vi "Find Average Center.vi"(5 "Position":i32, 7 "Tray Number":i32, 8 "Type of Hexaboard":T1, 9 "XYZTheta":dbl[](array[numeric]), 11 "Gantry In":refnum<k24>) -> (1 "XYZTheta":dbl[](array[numeric]) format="%.6g", 3 "Gantry Out":refnum<k24>)   [LabVIEW 2021, in "Component Tray.lvclass"]
uses:
  Component Tray.lvclass
  Find Component.ctl
  Controller/Camera/Machine Vision.ctl
  C:/Program Files (x86)/Aerotech/A3200/LabVIEW/2010/Bin/Aerotech.A3200.dll
  Program Files (x86)/Aerotech/A3200/LabVIEW/2010/Bin/Aerotech.A3200.dll
  Controller/Camera/Image processing.ctl
  Controller/Camera/Camera settings.ctl
  Controller/Camera/Material.ctl
  Routine/TypeOfHexaboard.ctl
  Controller/Camera/Edmund Optics/Edmund Optics.lvclass
  C:/Users/hep/Documents/UCSB-CMU-GantryCode/UCSB-Gantry-HEP-main (3)/UCSB-Gantry-HEP-main/Classes/Controller/Camera/Camera.lvclass
  Program Files (x86)/National Instruments/LabVIEW 2021/examples/Connectivity/Python/support/PythonVersionsEnum.ctl
  Controller/Camera/Camera.lvclass
  Controller/Motion/A3200/A3200.lvclass
  Controller/Motion/Motion.lvclass
  Routine/Routine.lvclass
panel:
  out "Program Stopped":bool
  out "XY Graph":cluster{"X":dbl, "Y":dbl}[](graph)
  out "Sensor ID Location":dbl[](array[numeric])
  in  "Go to Sensor ID":bool
  out "CH1 Location":dbl[](array[numeric])
  in  "Verify CH1":bool
  out "CH1 correct?":bool
  in  "Go to CH1":bool
  in  "Focus step size":dbl format="%#_13g"
  in  "number of focus steps":i32
  out "Average Strength":dbl
  in  "Focus":bool
  in  "Material":T2
  out "All fiducials recorded":bool
  in  "Override presets":bool
  in  "Camera settings":T3={"Gamma"=1.6, "Gain"=0, "Sharpness"=0, "Contrast"=0.0, "Exposure"=0.0078125} {"Exposure" min=0.000244140625 max=0.5 scale=0.0002..0.5; "Contrast" min=0.0 max=1.0 scale=0.001..1.0; "Sharpness" min=0 max=2 step=1 scale=0.0..2.0; "Gain" min=0 max=100 step=1 scale=0.1..100.0; "Gamma" min=0.01 max=10.0 scale=0.01..10.0}
  in  "Image processing":T4={"Brightness"=128.0, "Contrast"=45.0, "Gamma"=1.0471123} {"Brightness" scale=0.0..400.0; "Contrast" scale=0.0..90.0; "Gamma" scale=0.005..5.0}
  in  "Machine Vision":T5=enum."Sensor Fiducials"
  out "Gantry":dbl[](array[numeric]) format="%.6g"
  out "Sum":dbl[](array[numeric]) format="%.6g"
  out "Bottom Right XY":dbl[](array[numeric]) format="%.6g"
  out "Bottom Left XY":dbl[](array[numeric]) format="%.6g"
  out "Top Right XY":dbl[](array[numeric]) format="%.6g"
  out "Top Left XY":dbl[](array[numeric]) format="%.6g"
  in  "Record Bottom Left":bool
  in  "Record Bottom Right":bool
  in  "Record Top Right":bool
  in  "Record Top Left":bool
  in  "Go to Bottom Right":bool
  in  "Go to Bottom Left":bool
  in  "Go to Top Right":bool
  in  "Go to Top Left":bool
  in  "Joystick":bool
  out "Camera":dbl[](array[numeric]) format="%.6g"
  in  "Go to Center":bool
  in  "Component":T6
  in  "Stop Program":bool
  out "Image":T7(plugin-control)
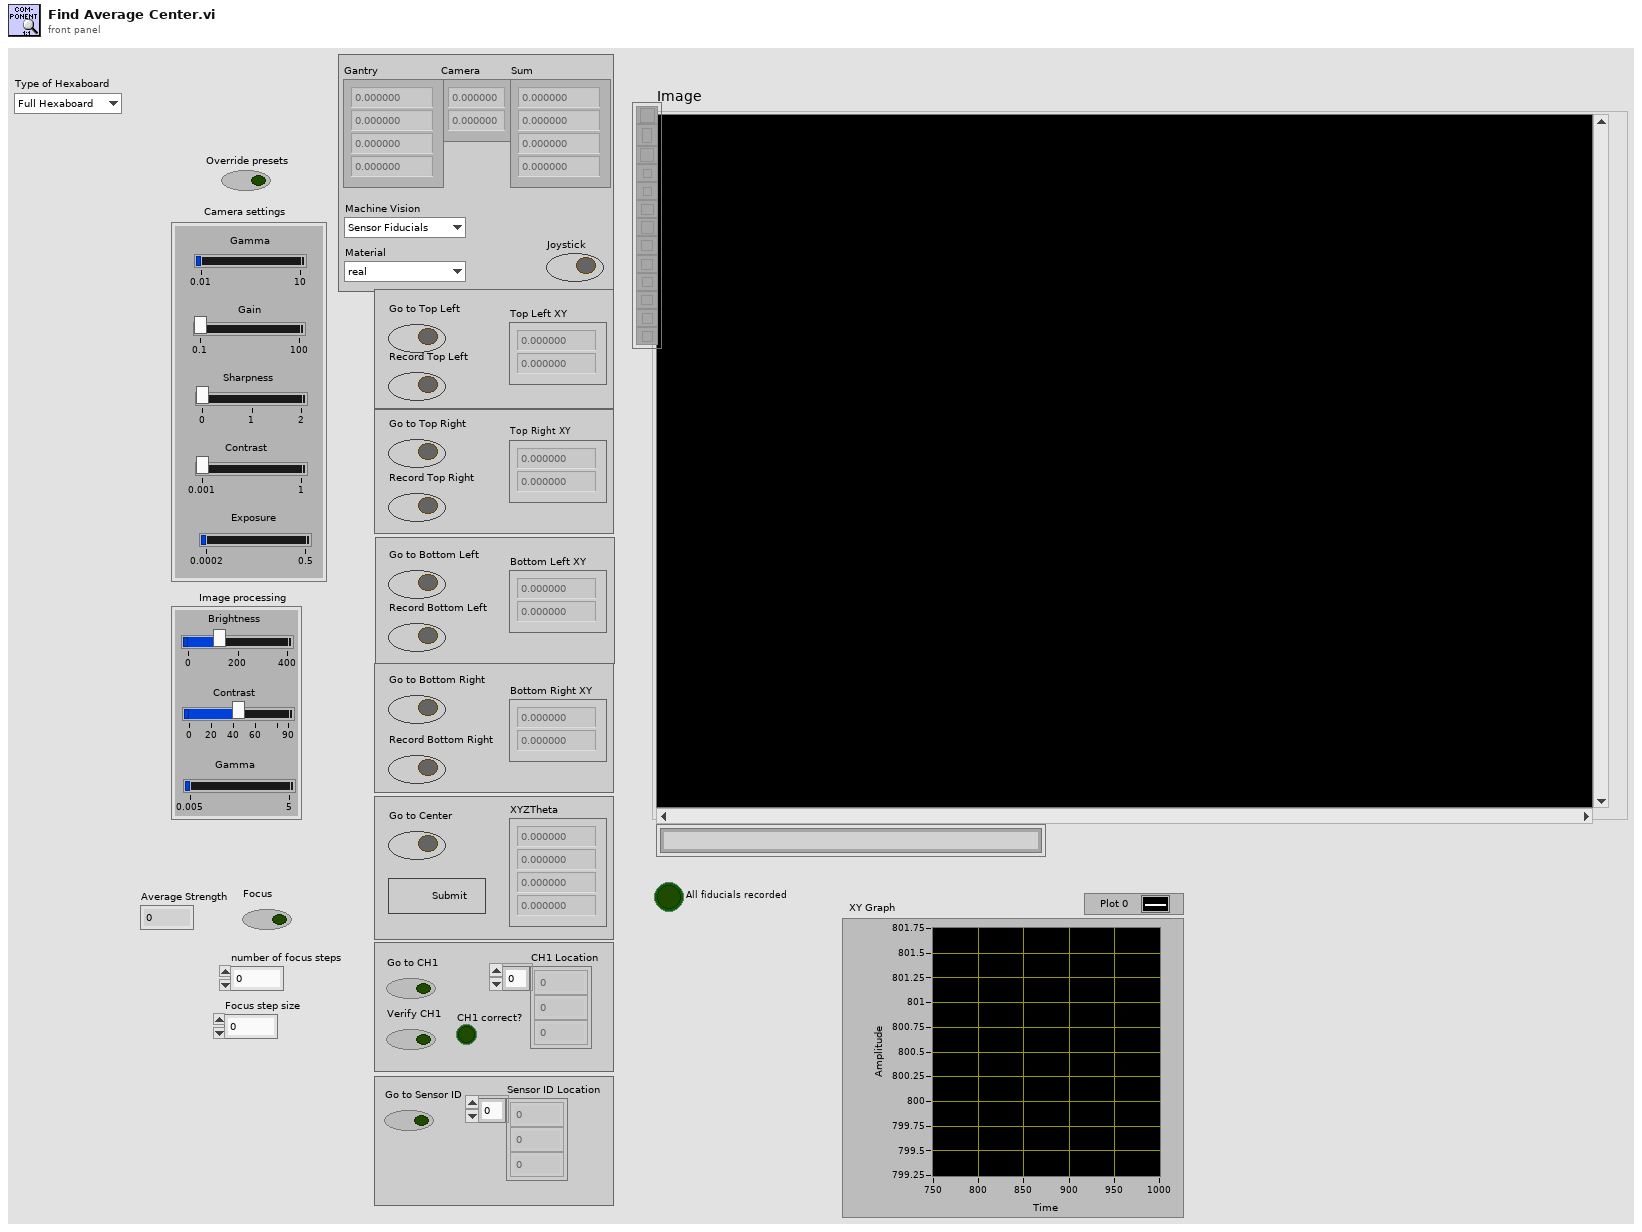
[diagram p1: front panel]
types:
  T1 = typedef "Routine.lvclass/TypeOfHexaboard.ctl" = enum16{"Full Hexaboard", "Right Partial PCB", "Right Partial Sensor", "Al Dummy Right Partial Sensor"}
  T2 = typedef "Camera.lvclass/Material.ctl" = enum16{"real", "dummy", "PETG"}
  T3 = typedef "Camera.lvclass/Camera settings.ctl" = cluster{"Gamma":dbl, "Gain":i64, "Sharpness":i64, "Contrast":dbl, "Exposure":dbl}
  T4 = typedef "Camera.lvclass/Image processing.ctl" = cluster{"Brightness":sgl, "Contrast":sgl, "Gamma":sgl}
  T5 = typedef "Camera.lvclass/Machine Vision.ctl" = enum16{"None", "Tray Fiducials", "Sensor Fiducials", "HPK Silicon", "Partial Hexaboard", "Partial Hexaboard Test", "100um dot", "Hexaboard", "Corner (TL, BR)", "Corner (BL, TR)", "V3 Sensor Cross", "V3 Sensor Circle"}
  T6 = typedef "Component Tray.lvclass/Find Component.ctl" = cluster{"New Fiducials":dbl[], "Past Fiducials":dbl[], "XYZTheta":dbl[], "Fiducials Path":path, "Position":i32, "CH1 Location":dbl[], "Sensor ID Location":dbl[]}
  T7 = typedef "IMAQ Image.ctl" = refnum<image>
  T8 = typedef "File Paths.ctl" = cluster{"Glue Pattern Folder":path, "Carrier Tray Folder":path, "Pick Up Tool Fixture Folder":path, "Components Folder":path, "Bellows Tool Offset.txt":path, "Pick Up Tool Offset.txt":path, "Dispense Tip Offset.txt":path, "Log Files":path, "Gantry Assembly Map.txt":path, "Syringe and offset map.txt":path}
  T9 = typedef "PythonVersionsEnum.ctl" = enum16{"3.6", "3.7", "3.8", "3.9"}
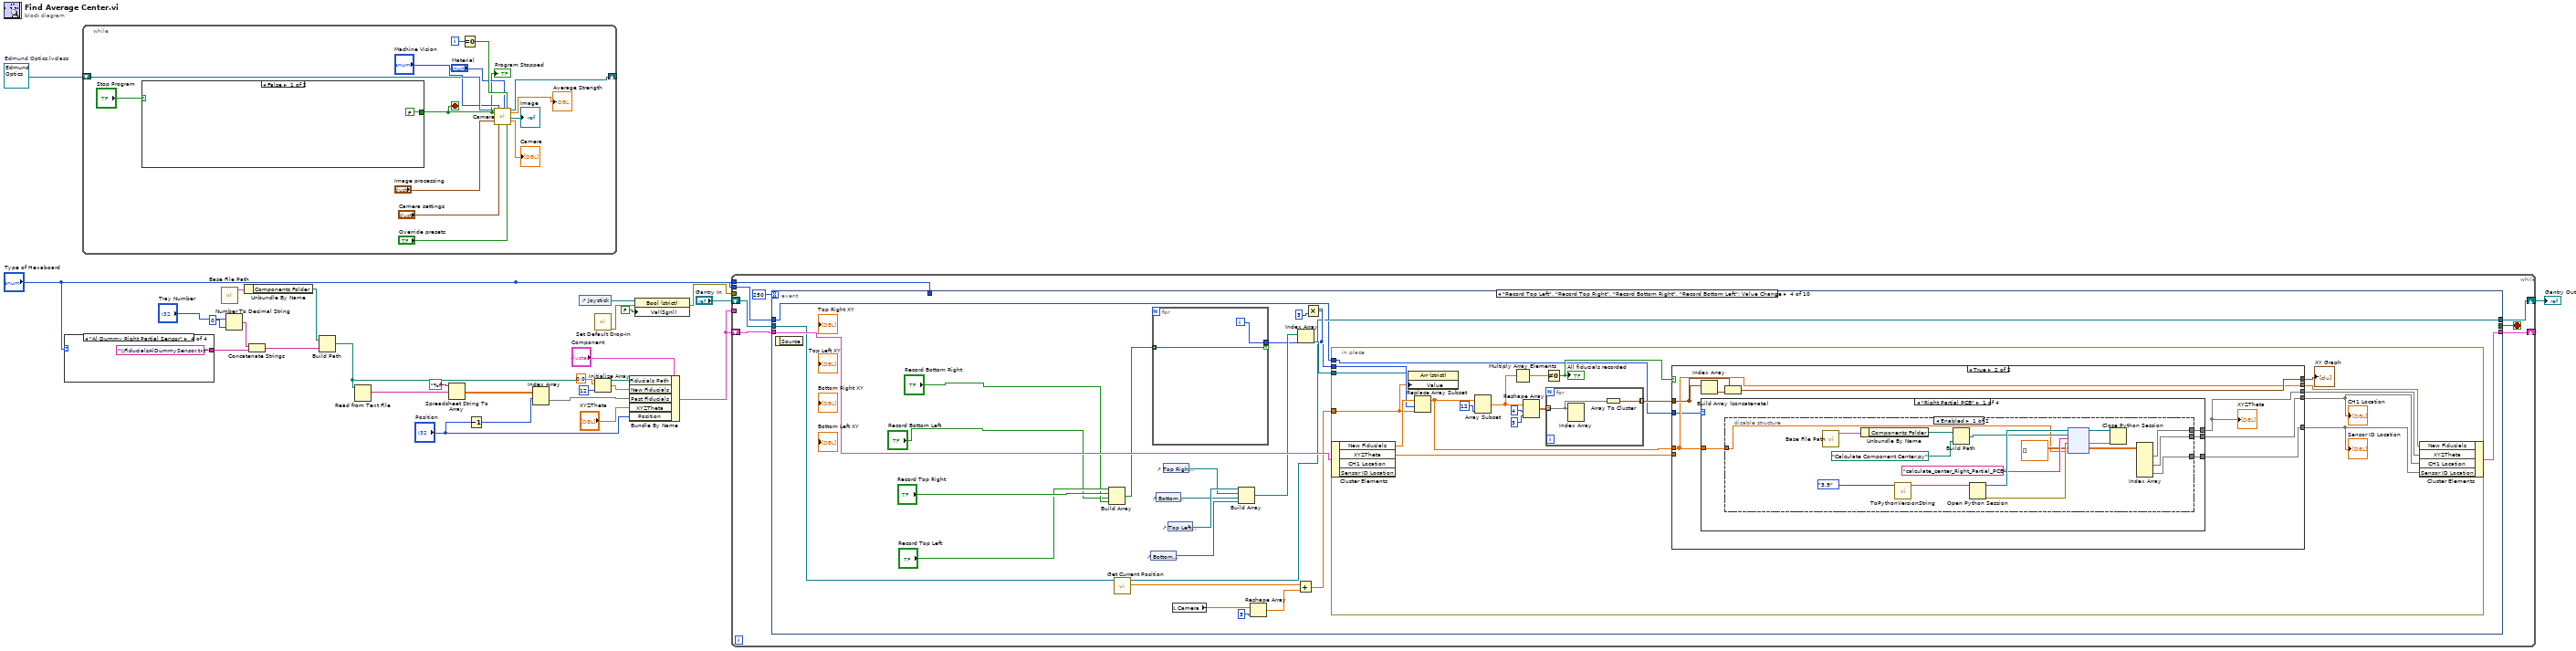
[diagram p0: block diagram]
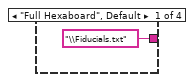
[diagram p2: hidden frame]
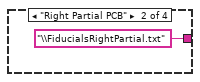
[diagram p3: hidden frame]
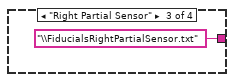
[diagram p4: hidden frame]
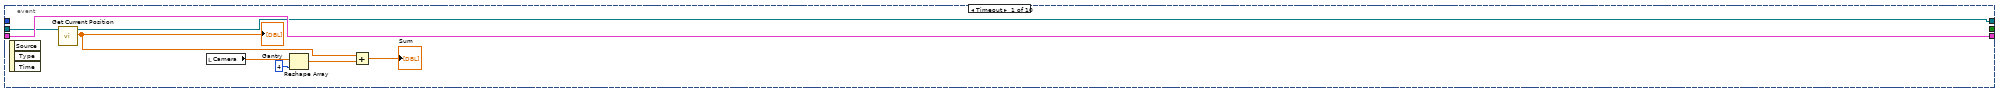
[diagram p5: hidden frame]
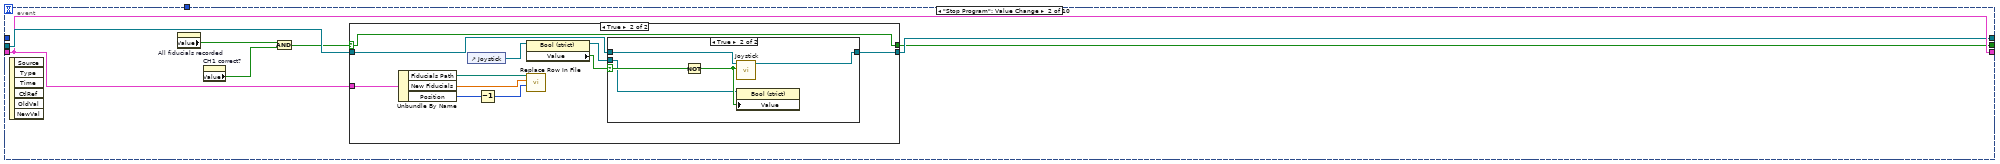
[diagram p6: hidden frame]
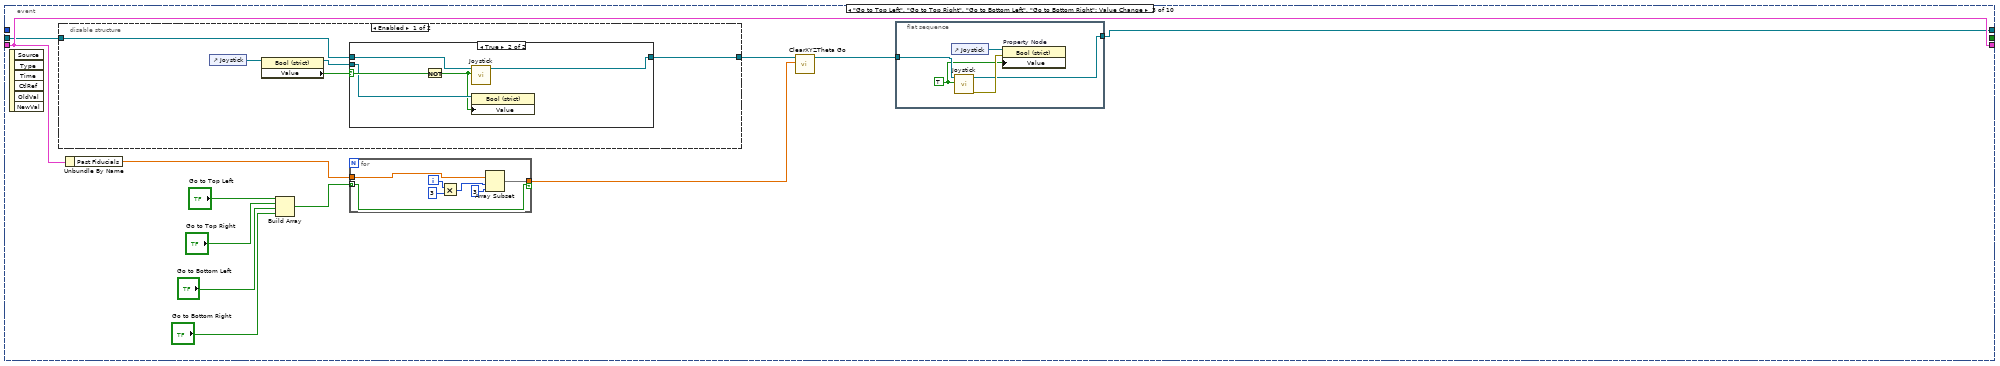
[diagram p9: hidden frame]
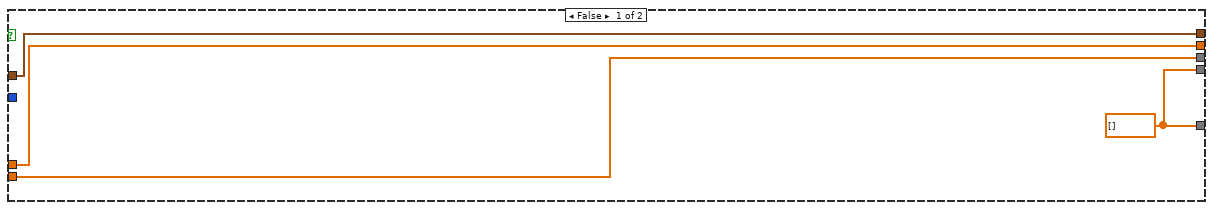
[diagram p12: hidden frame]
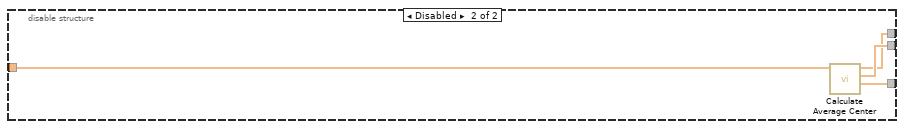
[diagram p13: hidden frame]
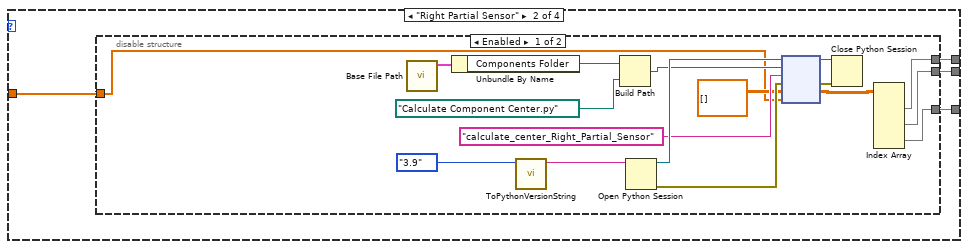
[diagram p14: hidden frame]
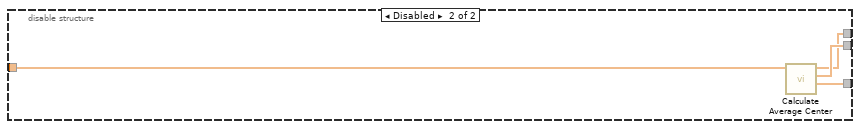
[diagram p15: hidden frame]
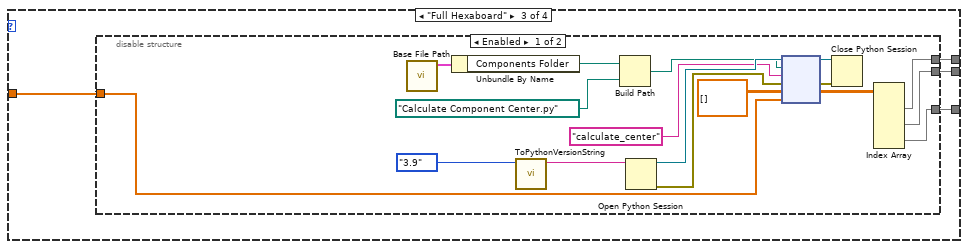
[diagram p16: hidden frame]
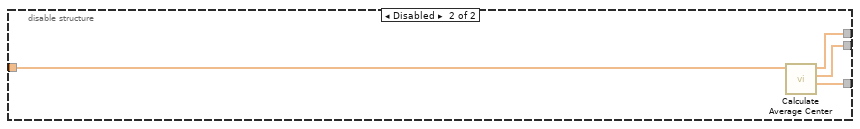
[diagram p17: hidden frame]
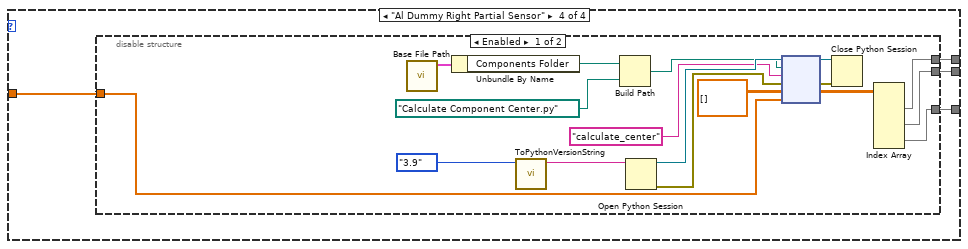
[diagram p18: hidden frame]
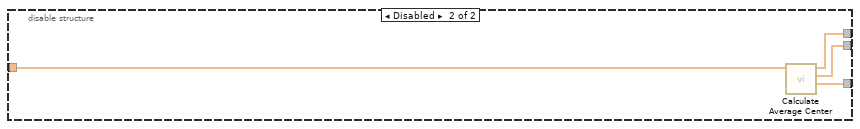
[diagram p19: hidden frame]
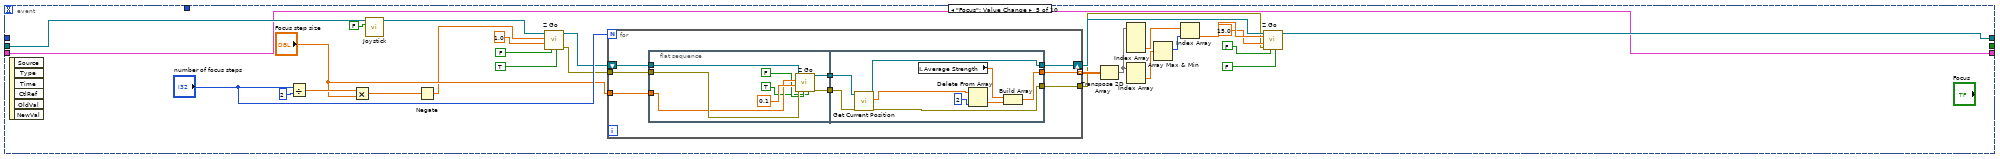
[diagram p20: hidden frame]
diagram:
  w24 = refnum<class "Edmund Optics.lvclass"> refnum  # Edmund Optics.lvclass
  n1 = case shown="\"Al Dummy Right Partial Sensor\"" "Type of Hexaboard" {
    tunnel: ["\\Fiducials.txt" ("string") "\\FiducialsRightPartial.txt" ("string") "\\FiducialsRightPartialSensor.txt" ("string") "\\FiducialsAlDummySensor.txt" ("string")] -> w19
    frame "Full Hexaboard", Default {
    }
    frame "Right Partial PCB" {
    }
    frame "Right Partial Sensor" {
    }
    frame "Al Dummy Right Partial Sensor" {
    }
  }
  n2 = while {
    shift-right: [w42] -> _
    shift-left: w24 -> [w46]
    i -> [w38]
    stop <- w33 stop-if-true
    n3 = case shown="False" "Stop Program" {
      tunnel: [FALSE w48] -> w33
      frame False {
      }
      frame True {
        n4 = property on="All fiducials recorded" class="Bool (strict)"() -> ("Value"=w51:bool)  [unwired: 2 in, 2 out]
        n5 = property on="CH1 correct?" class="Bool (strict)"() -> ("Value"=w49:bool)  [unwired: 2 in, 2 out]
        n6 = And(x=w51, y=w49) -> (x .and. y?=w50:bool)
        n7 = case shown="False" w50 {
          tunnel: [FALSE TRUE] -> w48
          frame False {
            n8 = One Button Dialog(message="At least one fiducial not recorded or component orientation not verified.") -> ()  [unwired: 1 in, 1 out]
          }
          frame True {
            n9 = property on="All fiducials recorded" class="Bool (strict)"("Val(Sgnl)"=FALSE) -> ()  [unwired: 2 in, 2 out]
          }
        }
      }
    }
    "Program Stopped" <- w33
    n10 = Equal To 0?(x=w38) -> (x = 0?=w37:bool)
    n11 = call "Camera.vi"("Camera in"=w46, "Stop"=w33, "BCG Image Processing"="Image processing", "Machine Vision"="Machine Vision", "Camera settings"="Camera settings", "Material"="Material", "Loop 0"=w37, "Override presets"="Override presets") -> ("Camera out"=w42:refnum<class "Edmund Optics.lvclass">, "Average Strength"=→"Average Strength":dbl, "Image"=→"Image":T7, "Camera"=→"Camera":dbl[])  [unwired: 5 in, 3 out]
  }
  n12 = call "Base File Path.vi"() -> ("Paths Out"=w15:T8)  [unwired: 11 in]
  n13 = Number To Decimal String(number="Tray Number", width (-)=i16 0) -> (decimal integer string=w18:string)
  n14 = Unbundle By Name(w15) -> ("Components Folder"=w17:path)
  n15 = Concatenate Strings "Concatenate Strings"(w18, w19) -> (w20:string)
  n16 = Build Path(base path=w17, name or relative path=w20) -> (appended path=w9:path)
  n17 = Read from Text File(file (use dialog)=w9) -> (text=w21:string)  [unwired: 3 in, 3 out]
  n18 = Spreadsheet String To Array(format string="%f", spreadsheet string=w21) -> (array=w23:dbl[][])  [unwired: 2 in]
  n19 = Decrement(x="Position") -> (x-1=w6:i32)
  n20 = Index Array "Index Array"(array=w23, index (row)=w6) -> (element=w13:dbl[])  [unwired: 1 in]
  n21 = control-ref of="Joystick"() -> (w27:refnum<vi>)
  n22 = Initialize Array(0.0 ("element"), 12 ("dimension size")) -> (w12:dbl[])
  n23 = call "Set Default Drop-In.vi"() -> ("error out"=w5:errorcluster)  [unwired: 11 in]
  n24 = Bundle By Name "Bundle By Name"(cluster="Component", "Fiducials Path"=w9, "New Fiducials"=w12, "Past Fiducials"=w13, "XYZTheta"="XYZTheta", "Position"="Position") -> (w2:T6)
  n25 = property class="Bool (strict)"(reference=w27, error in=w5, "Val(Sgnl)"=FALSE) -> (error out=w25:errorcluster)  [unwired: 1 out]
  n26 = while {
    shift-right: [w61] -> _
    shift-left: w2 -> [w62]
    tunnel: w25 -> [_]
    shift-right: [w58] -> w3
    shift-left: "Gantry In" -> [w59]
    tunnel: "Type of Hexaboard" -> [w57]
    tunnel: w2 -> [_]
    tunnel: "Type of Hexaboard" -> [w56]
    stop <- w63 stop-if-true
    n27 = event shown="[3] \"Record Top Left\", \"Record Top Right\", \"Record Bottom Right\", \"Record Bottom Left\": Value Change" {
      selector: _ -> [_ _ _ _ _ _ _ _ _ _]
      dyn-events: _ -> [_ _ _ _ _ _ _ _ _ _]
      timeout: 250 -> [_ _ _ _ _ _ _ _ _ _]
      tunnel: [_ w75 _ _ _ _ _ _ _ _] -> w63
      tunnel: w62 -> [w70 w77 w102 w156 w302 w348 w355 w370 w385 w395]
      tunnel: [w70 w77 w102 w155 w302 w348 w355 w370 w385 w395] -> w61
      tunnel: w59 -> [w66 w78 w101 w140 w304 w347 w351 w366 w381 w396]
      tunnel: [w65 w76 w98 w138 w303 w345 w349 w364 w379 w396] -> w58
      tunnel: w57 -> [_ _ _ w137 _ _ _ _ _ _]
      tunnel: w56 -> [_ _ _ _ _ _ _ _ _ _]
      event Timeout {
        n28 = event-data() -> ()  [unwired: 1 in, 3 out]
        n29 = call "Get Current Position.vi"("Gantry In"=w66) -> ("XYZTheta Out"=w64:dbl[], "Gantry Out"=w65:refnum<k24>)  [unwired: 8 in, 1 out]
        "Gantry" <- w64
        n30 = local read "Camera"() -> (w69:dbl[])
        n31 = Reshape Array(w69, 4 ("dimension size")) -> (w67:dbl[])
        n32 = Add(x=w64, y=w67) -> (x+y=→"Sum":dbl[])
      }
      event "Stop Program": Value Change {
        n33 = event-data() -> ()  [unwired: 1 in, 6 out]
        n34 = property on="All fiducials recorded" class="Bool (strict)"() -> ("Value"=w73:bool)  [unwired: 2 in, 2 out]
        n35 = property on="CH1 correct?" class="Bool (strict)"() -> ("Value"=w74:bool)  [unwired: 2 in, 2 out]
        n36 = And(x=w73, y=w74) -> (x .and. y?=w72:bool)
        n37 = case shown="True" w72 {
          selector: w72 -> [w79 w88]
          tunnel: w78 -> [w80 w90]
          tunnel: w77 -> [_ w91]
          tunnel: [w80 w89] -> w76
          tunnel: [w79 w88] -> w75
          frame False {
          }
          frame True {
            n38 = Unbundle By Name(w91) -> ("Fiducials Path"=w85:path, "New Fiducials"=w84:dbl[], "Position"=w86:i32)
            n39 = control-ref of="Joystick"() -> (w82:refnum<vi>)
            n40 = Decrement(x=w86) -> (x-1=w87:i32)
            n41 = property class="Bool (strict)"(reference=w82) -> (reference out=w81:refnum<vi>, "Value"=w83:bool)  [unwired: 1 in, 1 out]
            n42 = call "Replace Row In File.vi"("Index"=w87, "Insert Array"=w84, "Path"=w85) -> ()  [unwired: 8 in, 1 out]
            n43 = case shown="True" w83 {
              selector: w83 -> [_ w97]
              tunnel: w90 -> [w92 w96]
              tunnel: [w92 w95] -> w89
              tunnel: w81 -> [_ w93]
              frame False {
              }
              frame True {
                n44 = Not(x=w97) -> (.not. x?=w94:bool)
                n45 = call "Joystick.vi"("Joystick"=w94, "Gantry In"=w96) -> ("Gantry Out"=w95:refnum<k24>)  [unwired: 8 in, 1 out]
                n46 = property class="Bool (strict)"(reference=w93, "Value"=w94) -> ()  [unwired: 1 in, 2 out]
              }
            }
          }
        }
      }
      event "Go to Top Left", "Go to Top Right", "Go to Bottom Left", "Go to Bottom Right": Value Change {
        n47 = event-data() -> ()  [unwired: 1 in, 6 out]
        n48 = disable-structure shown="Enabled" {
          disable-tunnel: w101 -> [w112 _]
          disable-tunnel: [w111 _] -> w100
          frame Enabled {
            n49 = control-ref of="Joystick"() -> (w110:refnum<vi>)
            n50 = property class="Bool (strict)"(reference=w110) -> (reference out=w113:refnum<vi>, "Value"=w114:bool)  [unwired: 1 in, 1 out]
            n51 = case shown="True" w114 {
              selector: w114 -> [_ w120]
              tunnel: w112 -> [w115 w118]
              tunnel: [w115 w116] -> w111
              tunnel: w113 -> [_ w119]
              frame False {
              }
              frame True {
                n52 = Not(x=w120) -> (.not. x?=w117:bool)
                n53 = call "Joystick.vi"("Joystick"=w117, "Gantry In"=w118) -> ("Gantry Out"=w116:refnum<k24>)  [unwired: 8 in, 1 out]
                n54 = property class="Bool (strict)"(reference=w119, "Value"=w117) -> ()  [unwired: 1 in, 2 out]
              }
            }
          }
          frame Disabled {
          }
        }
        n55 = Unbundle By Name(w102) -> ("Past Fiducials"=w104:dbl[])
        n56 = Build Array("Go to Top Left", "Go to Top Right", "Go to Bottom Left", "Go to Bottom Right") -> (w105:bool[])
        n57 = for {
          tunnel: w105 -> [w132] mode=indexing
          tunnel: w104 -> [w131]
          tunnel: [w126] -> w103 if=w132
          i -> [w129]
          n58 = Multiply(x=w129, y=3) -> (x*y=w127:i32)
          n59 = Array Subset(array=w131, index=w127, length=3) -> (w126:dbl[])
        }
        n60 = call "ClearXYZTheta Go.vi"("XYZTheta In"=w103, "Gantry In"=w100) -> ("Gantry Out"=w99:refnum<k24>)  [unwired: 7 in, 2 out]
        n61 = flat-sequence {
          tunnel: w99 -> [w125]
          tunnel: [w122] -> w98
          frame #0 {
            w121 = TRUE
            n62 = control-ref of="Joystick"() -> (w124:refnum<vi>)
            n63 = call "Joystick.vi"("Joystick"=w121, "Gantry In"=w125) -> ("error out"=w123:errorcluster, "Gantry Out"=w122:refnum<k24>)  [unwired: 8 in]
            n64 = property on="Property Node" class="Bool (strict)"(reference=w124, error in=w123, "Value"=w121) -> ()  [unwired: 2 out]
          }
        }
      }
      event "Record Top Left", "Record Top Right", "Record Bottom Right", "Record Bottom Left": Value Change {
        n65 = event-data() -> ()  [unwired: 1 in, 1 out]
        n66 = Build Array("Record Top Left", "Record Top Right", "Record Bottom Left", "Record Bottom Right") -> (w154:bool[])
        n67 = call "Get Current Position.vi"("Gantry In"=w140) -> ("XYZTheta Out"=w139:dbl[], "Gantry Out"=w138:refnum<k24>)  [unwired: 8 in, 1 out]
        n68 = control-ref of="Bottom Right XY"() -> (w150:refnum<vi>)
        n69 = for {
          tunnel: w154 -> [w157] mode=indexing
          tunnel: [w158] -> w146 if=w157
          i -> [w158]
        }
        n70 = control-ref of="Bottom Left XY"() -> (w151:refnum<vi>)
        n71 = control-ref of="Top Right XY"() -> (w152:refnum<vi>)
        n72 = control-ref of="Top Left XY"() -> (w153:refnum<vi>)
        n73 = local read "Camera"() -> (w143:dbl[])
        n74 = Build Array(w153, w152, w151, w150) -> (w149:refnum<vi>[])
        n75 = Reshape Array(w143, 3 ("dimension size")) -> (w142:dbl[])
        n76 = Add(x=w139, y=w142) -> (x+y=w141:dbl[])
        n77 = Index Array(array=w149, index=w146) -> (element=w148:refnum<vi>)
        n78 = Multiply(x=w146, y=3) -> (x*y=w144:i32)
        n79 = in-place {
          in-place-border: w144 -> [w176]
          in-place-border: w148 -> [w174]
          in-place-border: w141 -> [w172]
          in-place-border: w137 -> [w159]
          n80 = in-place-cluster #1(w156) -> ("New Fiducials"=w177:dbl[], "XYZTheta"=w173:dbl[])  [unwired: 2 out]
          n81 = property class="Arr (strict)"(reference=w174, "Value"=w172) -> ()  [unwired: 1 in, 2 out]
          n82 = Replace Array Subset(array=w177, new element=w172, index=w176) -> (w171:dbl[])
          n83 = Array Subset(array=w171, length=12) -> (w166:dbl[])  [unwired: 1 in]
          n84 = Multiply Array Elements(1:w166) -> (0:w169:dbl)
          n85 = Reshape Array(w166, 4 ("dimension size"), 3 ("dimension size")) -> (w163:dbl[][])
          n86 = Not Equal To 0?(x=w169) -> (x != 0?=w160:bool)
          "All fiducials recorded" <- w160
          n87 = for {
            tunnel: w163 -> [w179] mode=indexing
            tunnel: [w180] -> w162 mode=indexing
            n88 = Index Array(array=w179) -> ()  [unwired: 2 in, 2 out]
            n89 = Array To Cluster(array=w179) -> (cluster=w180:cluster{"[0]":dbl, "[1]":dbl})
          }
          n90 = case shown="True" w160 {
            tunnel: [w183 w186] -> w178
            tunnel: w171 -> [w184 w189]
            tunnel: [w184 w189] -> w175
            tunnel: w173 -> [w183 _]
            tunnel: [w182 w187] -> w168
            tunnel: [w182 w188] -> w167
            tunnel: w162 -> [w181 w192]
            tunnel: [w181 w190] -> w161
            tunnel: w159 -> [_ w185]
            frame False {
              w182 = dbl[] [] ("CH1 location")
            }
            frame True {
              n91 = Index Array(array=w192) -> (element=w191:cluster{"[0]":dbl, "[1]":dbl})  [unwired: 1 in]
              n92 = case shown="\"Right Partial PCB\"" w185 {
                tunnel: w189 -> [w196 w221 w246 w271]
                tunnel: [w195 w220 w245 w270] -> w188
                tunnel: [w194 w219 w244 w269] -> w187
                tunnel: [w193 w218 w243 w268] -> w186
                frame "Right Partial PCB" {
                  n93 = disable-structure shown="Enabled" {
                    disable-tunnel: w196 -> [w201 w214]
                    disable-tunnel: [w197 w217] -> w195
                    disable-tunnel: [w198 w216] -> w194
                    disable-tunnel: [w199 w215] -> w193
                    frame Enabled {
                      n94 = call "Base File Path.vi"() -> ("Paths Out"=w206:T8)  [unwired: 11 in]
                      n95 = Unbundle By Name(w206) -> ("Components Folder"=w204:path)
                      n96 = call "ToPythonVersionString.vi"("python version"=PythonVersionsEnum."3.9") -> ("python version string"=w212:string)  [unwired: 10 in]
                      n97 = Build Path(base path=w204, name or relative path=path "Calculate Component Center.py") -> (appended path=w203:path)
                      n98 = Open Python Session(python version=w212) -> (session out=w211:refnum<k35>, error out=w209:errorcluster)  [unwired: 2 in]
                      n99 = node(w211, w203, "calculate_center_Right_Partial_PCB" ("function name"), w209, dbl[][] [], w201) -> (w210:refnum<k35>, w208:errorcluster, w200:dbl[][])  [unwired: 1 in, 2 out]
                      n100 = Close Python Session(session in=w210, error in=w208) -> ()  [unwired: 1 out]
                      n101 = Index Array "Index Array"(array=w200) -> (element #1=w199:dbl[], element #2=w198:dbl[], element #3=w197:dbl[])  [unwired: 6 in]
                    }
                    frame Disabled {
                      n102 = call "Calculate Average Center.vi"("Gantry Fiducials"=w214) -> ("Sensor ID Location"=w217:dbl[], "CH1 Location"=w216:dbl[], "XYZTheta"=w215:dbl[])  [unwired: 8 in]
                    }
                  }
                }
                frame "Right Partial Sensor" {
                  n103 = disable-structure shown="Enabled" {
                    disable-tunnel: w221 -> [w226 w239]
                    disable-tunnel: [w222 w242] -> w220
                    disable-tunnel: [w223 w241] -> w219
                    disable-tunnel: [w224 w240] -> w218
                    frame Enabled {
                      n104 = call "Base File Path.vi"() -> ("Paths Out"=w231:T8)  [unwired: 11 in]
                      n105 = Unbundle By Name(w231) -> ("Components Folder"=w229:path)
                      n106 = call "ToPythonVersionString.vi"("python version"=PythonVersionsEnum."3.9") -> ("python version string"=w237:string)  [unwired: 10 in]
                      n107 = Build Path(base path=w229, name or relative path=path "Calculate Component Center.py") -> (appended path=w228:path)
                      n108 = Open Python Session(python version=w237) -> (session out=w236:refnum<k35>, error out=w234:errorcluster)  [unwired: 2 in]
                      n109 = node(w236, w228, "calculate_center_Right_Partial_Sensor" ("function name"), w234, dbl[][] [], w226) -> (w235:refnum<k35>, w233:errorcluster, w225:dbl[][])  [unwired: 1 in, 2 out]
                      n110 = Close Python Session(session in=w235, error in=w233) -> ()  [unwired: 1 out]
                      n111 = Index Array(array=w225) -> (element #1=w224:dbl[], element #2=w223:dbl[], element #3=w222:dbl[])  [unwired: 6 in]
                    }
                    frame Disabled {
                      n112 = call "Calculate Average Center.vi"("Gantry Fiducials"=w239) -> ("Sensor ID Location"=w242:dbl[], "CH1 Location"=w241:dbl[], "XYZTheta"=w240:dbl[])  [unwired: 8 in]
                    }
                  }
                }
                frame "Full Hexaboard" {
                  n113 = disable-structure shown="Enabled" {
                    disable-tunnel: w246 -> [w251 w264]
                    disable-tunnel: [w247 w267] -> w245
                    disable-tunnel: [w248 w266] -> w244
                    disable-tunnel: [w249 w265] -> w243
                    frame Enabled {
                      n114 = call "Base File Path.vi"() -> ("Paths Out"=w256:T8)  [unwired: 11 in]
                      n115 = Unbundle By Name(w256) -> ("Components Folder"=w254:path)
                      n116 = call "ToPythonVersionString.vi"("python version"=PythonVersionsEnum."3.9") -> ("python version string"=w262:string)  [unwired: 10 in]
                      n117 = Build Path(base path=w254, name or relative path=path "Calculate Component Center.py") -> (appended path=w253:path)
                      n118 = Open Python Session(python version=w262) -> (session out=w261:refnum<k35>, error out=w259:errorcluster)  [unwired: 2 in]
                      n119 = node(w261, w253, "calculate_center" ("function name"), w259, dbl[][] [], w251) -> (w260:refnum<k35>, w258:errorcluster, w250:dbl[][])  [unwired: 1 in, 2 out]
                      n120 = Close Python Session(session in=w260, error in=w258) -> ()  [unwired: 1 out]
                      n121 = Index Array(array=w250) -> (element #1=w249:dbl[], element #2=w248:dbl[], element #3=w247:dbl[])  [unwired: 6 in]
                    }
                    frame Disabled {
                      n122 = call "Calculate Average Center.vi"("Gantry Fiducials"=w264) -> ("Sensor ID Location"=w267:dbl[], "CH1 Location"=w266:dbl[], "XYZTheta"=w265:dbl[])  [unwired: 8 in]
                    }
                  }
                }
                frame "Al Dummy Right Partial Sensor" {
                  n123 = disable-structure shown="Enabled" {
                    disable-tunnel: w271 -> [w276 w289]
                    disable-tunnel: [w272 w292] -> w270
                    disable-tunnel: [w273 w291] -> w269
                    disable-tunnel: [w274 w290] -> w268
                    frame Enabled {
                      n124 = call "Base File Path.vi"() -> ("Paths Out"=w281:T8)  [unwired: 11 in]
                      n125 = Unbundle By Name(w281) -> ("Components Folder"=w279:path)
                      n126 = call "ToPythonVersionString.vi"("python version"=PythonVersionsEnum."3.9") -> ("python version string"=w287:string)  [unwired: 10 in]
                      n127 = Build Path(base path=w279, name or relative path=path "Calculate Component Center.py") -> (appended path=w278:path)
                      n128 = Open Python Session(python version=w287) -> (session out=w286:refnum<k35>, error out=w284:errorcluster)  [unwired: 2 in]
                      n129 = node(w286, w278, "calculate_center" ("function name"), w284, dbl[][] [], w276) -> (w285:refnum<k35>, w283:errorcluster, w275:dbl[][])  [unwired: 1 in, 2 out]
                      n130 = Close Python Session(session in=w285, error in=w283) -> ()  [unwired: 1 out]
                      n131 = Index Array(array=w275) -> (element #1=w274:dbl[], element #2=w273:dbl[], element #3=w272:dbl[])  [unwired: 6 in]
                    }
                    frame Disabled {
                      n132 = call "Calculate Average Center.vi"("Gantry Fiducials"=w289) -> ("Sensor ID Location"=w292:dbl[], "CH1 Location"=w291:dbl[], "XYZTheta"=w290:dbl[])  [unwired: 8 in]
                    }
                  }
                }
              }
              "XYZTheta" <- w186
              n133 = Build Array (concatenate)(w192, w191) -> (w190:cluster{"[0]":dbl, "[1]":dbl}[])
            }
          }
          "CH1 Location" <- w168
          "Sensor ID Location" <- w167
          "XY Graph" <- w161
          n134 = in-place-cluster #1("New Fiducials"=w175, "XYZTheta"=w178, "CH1 Location"=w168, "Sensor ID Location"=w167) -> (w155:T6)
        }
      }
      event "Focus": Value Change {
        n135 = event-data() -> ()  [unwired: 1 in, 6 out]
        n136 = Divide(x="number of focus steps", y=2) -> (x/y=w307:dbl)
        n137 = Multiply(x=w307, y="Focus step size") -> (x*y=w305:dbl)
        n138 = call "Joystick.vi"("Joystick"=FALSE, "Gantry In"=w304) -> ("Gantry Out"=w298:refnum<k24>)  [unwired: 8 in, 1 out]
        n139 = Negate(x=w305) -> (-x=w299:dbl)
        n140 = call "Z Go.vi"("Increment"=TRUE, "Return Immediately"=FALSE ("Increment"), "Speed In"=1.0 ("Speed"), "Position In"=w299, "Gantry In"=w298) -> ("error out"=w296:errorcluster, "Gantry Out"=w297:refnum<k24>)  [unwired: 3 in, 2 out]
        n141 = for {
          N: "number of focus steps" -> [_]
          tunnel: [w324] -> w318 mode=indexing
          tunnel: w296 -> [w323]
          tunnel: [w321] -> w311
          shift-right: [w325] -> w312
          shift-left: w297 -> [w327]
          tunnel: "Focus step size" -> [w320]
          n142 = flat-sequence {
            tunnel: w327 -> [w335]
            tunnel: [w334] -> w326
            tunnel: w323 -> [w333]
            tunnel: [w332] -> w322
            tunnel: w320 -> [w330]
            tunnel: w326 -> [w344]
            tunnel: [w343] -> w325
            tunnel: [w342] -> w324
            tunnel: w322 -> [w338]
            tunnel: [w337] -> w321
            frame #0 {
              n143 = call "Z Go.vi"("Increment"=TRUE, "Return Immediately"=FALSE ("Increment"), "error in (no error)"=w333, "Speed In"=0.1 ("Speed"), "Position In"=w330, "Gantry In"=w335) -> ("error out"=w332:errorcluster, "Gantry Out"=w334:refnum<k24>)  [unwired: 2 in, 2 out]
            }
            frame #1 {
              n144 = call "Get Current Position.vi"("error in (no error)"=w338, "Gantry In"=w344) -> ("error out"=w337:errorcluster, "XYZTheta Out"=w341:dbl[], "Gantry Out"=w343:refnum<k24>)  [unwired: 7 in]
              n145 = local read "Average Strength"() -> (w336:dbl)
              n146 = Delete From Array(array=w341, index=2) -> (deleted portion=w339:dbl)  [unwired: 1 in, 1 out]
              n147 = Build Array(w336, w339) -> (w342:dbl[])
            }
          }
        }
        n148 = Transpose 2D Array(2D array=w318) -> (transposed array=w317:dbl[][])
        n149 = Index Array(array=w317) -> (element #2=w316:dbl[])  [unwired: 4 in, 1 out]
        n150 = Index Array(array=w317) -> (element=w319:dbl[])  [unwired: 2 in]
        n151 = Array Max & Min(array=w319) -> (max index (indices)=w315:i32)  [unwired: 3 out]
        n152 = Index Array(array=w316, index=w315) -> (element=w314:dbl)
        n153 = call "Z Go.vi"("Increment"=FALSE, "Return Immediately"=FALSE ("Increment"), "error in (no error)"=w311, "Speed In"=15.0 ("Speed"), "Position In"=w314, "Gantry In"=w312) -> ("Gantry Out"=w303:refnum<k24>)  [unwired: 2 in, 3 out]
      }
      event "Joystick": Value Change {
        n154 = event-data() -> ()  [unwired: 1 in, 6 out]
        n155 = call "Joystick.vi"("Joystick"="Joystick", "Gantry In"=w347) -> ("Gantry Out"=w345:refnum<k24>)  [unwired: 8 in, 1 out]
      }
      event "Go to Center": Value Change {
        n156 = event-data() -> ()  [unwired: 1 in, 6 out]
        n157 = Unbundle By Name(w355) -> ("XYZTheta"=w356:dbl[])
        n158 = control-ref of="Joystick"() -> (w352:refnum<vi>)
        n159 = property class="Bool (strict)"(reference=w352) -> (reference out=w353:refnum<vi>, "Value"=w354:bool)  [unwired: 1 in, 1 out]
        n160 = case shown="True" w354 {
          selector: w354 -> [_ w363]
          tunnel: w351 -> [w357 w360]
          tunnel: [w357 w359] -> w350
          tunnel: w353 -> [_ w362]
          frame False {
          }
          frame True {
            n161 = Not(x=w363) -> (.not. x?=w358:bool)
            n162 = call "Joystick.vi"("Joystick"=w358, "Gantry In"=w360) -> ("error out"=w361:errorcluster, "Gantry Out"=w359:refnum<k24>)  [unwired: 8 in]
            n163 = property class="Bool (strict)"(reference=w362, error in=w361, "Value"=w358) -> ()  [unwired: 2 out]
          }
        }
        n164 = call "ClearXYZTheta Go.vi"("XYZTheta In"=w356, "Gantry In"=w350) -> ("Gantry Out"=w349:refnum<k24>)  [unwired: 7 in, 2 out]
      }
      event "Go to CH1": Value Change {
        n165 = event-data() -> ()  [unwired: 1 in, 6 out]
        n166 = Unbundle By Name(w370) -> ("CH1 Location"=w371:dbl[])
        n167 = control-ref of="Joystick"() -> (w367:refnum<vi>)
        n168 = property class="Bool (strict)"(reference=w367) -> (reference out=w368:refnum<vi>, "Value"=w369:bool)  [unwired: 1 in, 1 out]
        n169 = case shown="True" w369 {
          selector: w369 -> [_ w378]
          tunnel: w366 -> [w372 w375]
          tunnel: [w372 w374] -> w365
          tunnel: w368 -> [_ w377]
          frame False {
          }
          frame True {
            n170 = Not(x=w378) -> (.not. x?=w373:bool)
            n171 = call "Joystick.vi"("Joystick"=w373, "Gantry In"=w375) -> ("error out"=w376:errorcluster, "Gantry Out"=w374:refnum<k24>)  [unwired: 8 in]
            n172 = property class="Bool (strict)"(reference=w377, error in=w376, "Value"=w373) -> ()  [unwired: 2 out]
          }
        }
        n173 = call "ClearXYZTheta Go.vi"("XYZTheta In"=w371, "Gantry In"=w365) -> ("Gantry Out"=w364:refnum<k24>)  [unwired: 7 in, 2 out]
      }
      event "Go to Sensor ID": Value Change {
        n174 = event-data() -> ()  [unwired: 1 in, 6 out]
        n175 = Unbundle By Name(w385) -> ("Sensor ID Location"=w386:dbl[])
        n176 = control-ref of="Joystick"() -> (w382:refnum<vi>)
        n177 = property class="Bool (strict)"(reference=w382) -> (reference out=w383:refnum<vi>, "Value"=w384:bool)  [unwired: 1 in, 1 out]
        n178 = case shown="True" w384 {
          selector: w384 -> [_ w393]
          tunnel: w381 -> [w387 w390]
          tunnel: [w387 w389] -> w380
          tunnel: w383 -> [_ w392]
          frame False {
          }
          frame True {
            n179 = Not(x=w393) -> (.not. x?=w388:bool)
            n180 = call "Joystick.vi"("Joystick"=w388, "Gantry In"=w390) -> ("error out"=w391:errorcluster, "Gantry Out"=w389:refnum<k24>)  [unwired: 8 in]
            n181 = property class="Bool (strict)"(reference=w392, error in=w391, "Value"=w388) -> ()  [unwired: 2 out]
          }
        }
        n182 = call "ClearXYZTheta Go.vi"("XYZTheta In"=w386, "Gantry In"=w380) -> ("Gantry Out"=w379:refnum<k24>)  [unwired: 7 in, 2 out]
      }
      event "Verify CH1": Value Change {
        n183 = event-data() -> ()  [unwired: 1 in, 6 out]
        "CH1 correct?" <- TRUE
      }
    }
  }
  "Gantry Out" <- w3
